vi "Shooter Speeds LUT.vi"(11 "Shooter States":T1) -> (3 "Target Velocity":dbl)   [LabVIEW 2015]
uses:
  Typedefs/Shooter States.ctl
  Gensubs/Bert_or_Ernie.vi
panel:
  in  "Pract. Bot Shooter LUT":dbl[](array[numeric])
  in  "Comp. Bot Shooter LUT":dbl[](array[numeric])
  # "all in rpm"
  # "off"
  # "off"
  # "close"
  # "close"
  # "far"
  # "far"
  # "intermediate"
  # "intermediate"
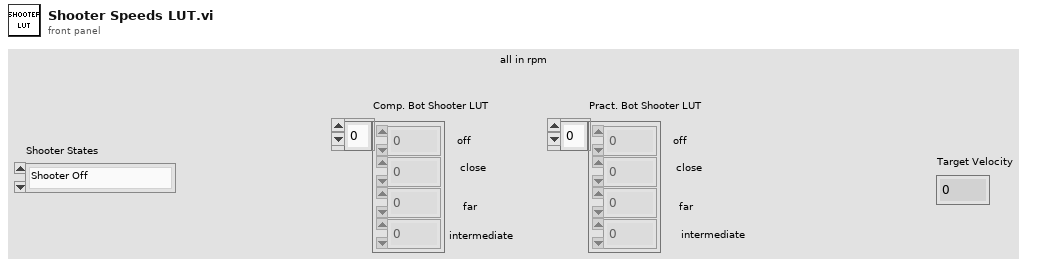
[diagram p1: front panel]
types:
  T1 = typedef "Shooter States.ctl" = enum16{"Shooter Off", "Shooter Far", "Shooter Close", "Shooter Intermediate"}
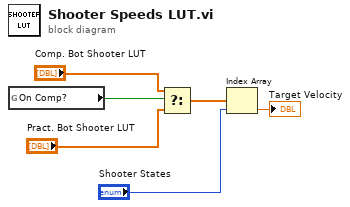
[diagram p0: block diagram]
diagram:
  n1 = global read "Bert_or_Ernie.vi" "On Comp?"() -> (w6:bool)
  n2 = Select(t="Comp. Bot Shooter LUT", s=w6, f="Pract. Bot Shooter LUT") -> (s? t:f=w3:dbl[])
  n3 = Index Array(array=w3, index="Shooter States") -> (element=→"Target Velocity":dbl)
